vi "Acc_X.vi"(1 "x_ini":dbl) -> (0 "x_Acc":dbl)   [LabVIEW 2010]
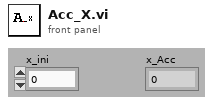
[diagram p1: front panel]
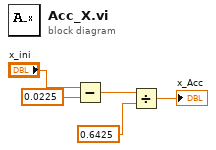
[diagram p0: block diagram]
diagram:
  n1 = Subtract(x="x_ini", y=0.0225) -> (x-y=w3:dbl)
  n2 = Divide(x=w3, y=0.6425) -> (x/y=→"x_Acc":dbl)
